vi "Drive Train Motion Track.vi"(6 "Ka":dbl, 7 "PID Settings":T2, 9 "Use Ave":bool, 10 "Array":T1(array[cluster]), 11 "Kv":dbl) -> ()   [LabVIEW 2015]
uses:
  Support/LightningPID Settings.ctl
panel:
  out "Right Velocity Chart":cluster{"left":dbl, "Rate":dbl}(graph)
  out "Right Distance Chart":cluster{"left":dbl, "Rate":dbl}(graph)
  out "Moter Power":cluster{"left":dbl, "Rate":dbl}(graph)
  out "Left Velocity Chart":cluster{"left":dbl, "Rate":dbl}(graph)
  out "Left Distance Chart":cluster{"left":dbl, "Rate":dbl}(graph)
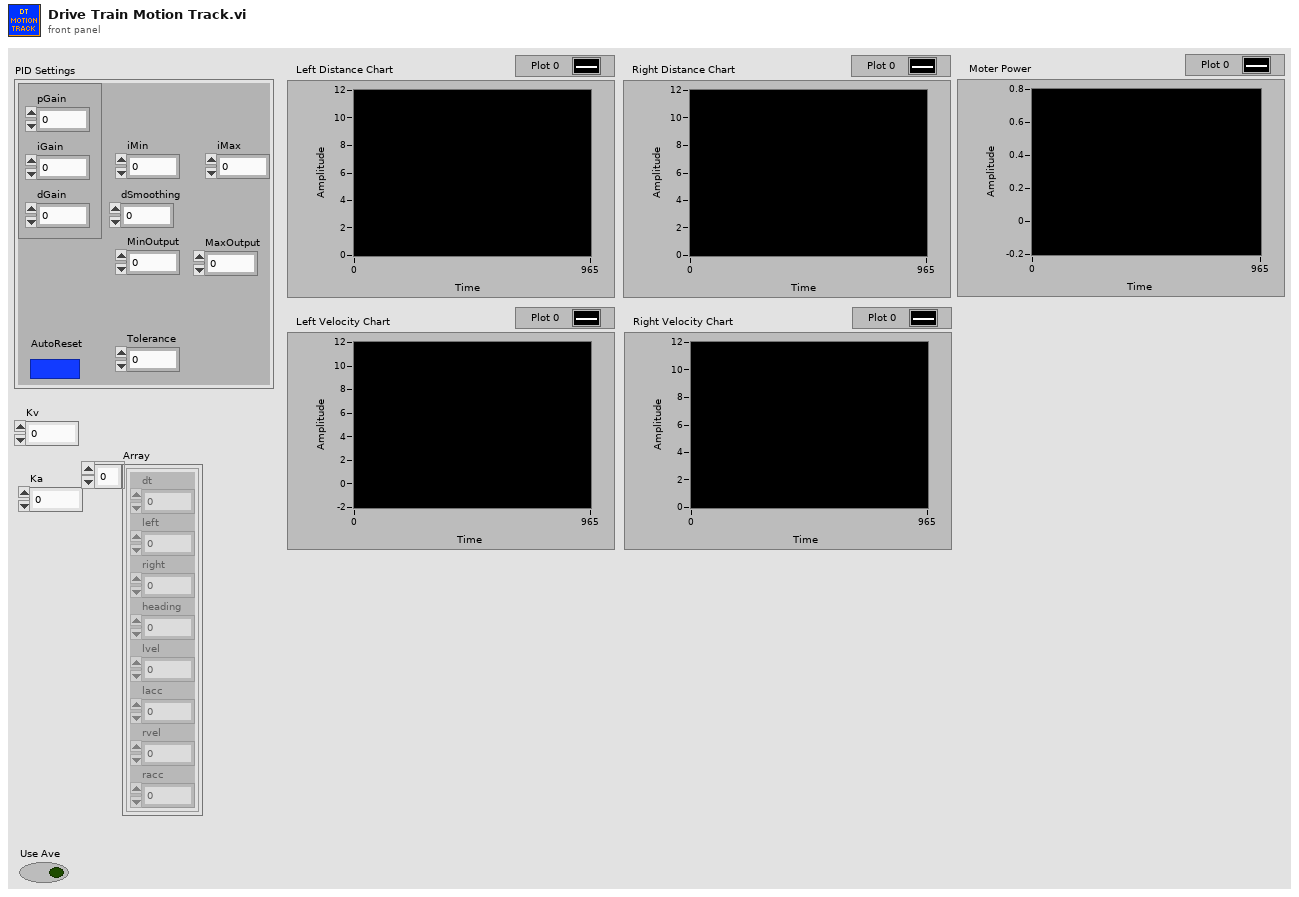
[diagram p1: front panel]
types:
  T1 = cluster{"dt":dbl, "left":dbl, "right":dbl, "heading":dbl, "lvel":dbl, "lacc":dbl, "rvel":dbl, "racc":dbl}[]
  T2 = typedef "LightningPID Settings.ctl" = cluster{"iMax":dbl, "iMin":dbl, "iGain":dbl, "pGain":dbl, "dGain":dbl, "MaxOutput":dbl, "MinOutput":dbl, "AutoReset":bool, "Tolerance":dbl, "dSmoothing":dbl}
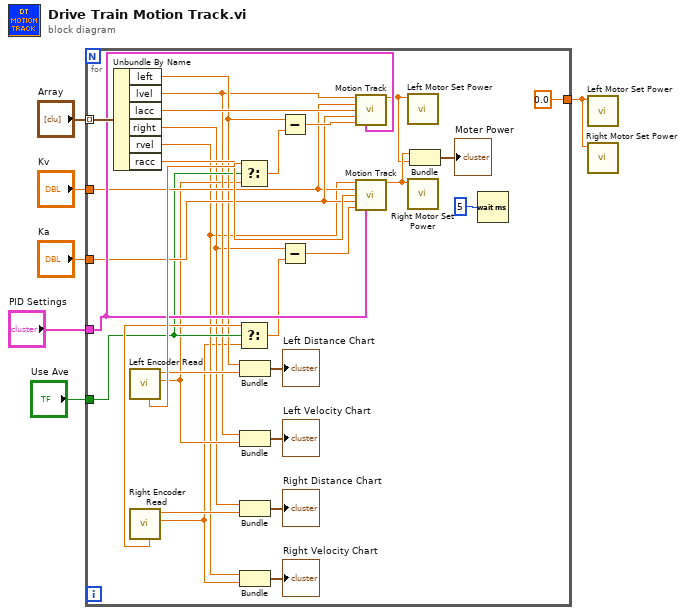
[diagram p0: block diagram]
diagram:
  n1 = for {
    tunnel: "Array" -> [w35] mode=indexing
    tunnel: [0.0] -> w2
    tunnel: "PID Settings" -> [w27]
    tunnel: "Ka" -> [w26]
    tunnel: "Kv" -> [w25]
    tunnel: "Use Ave" -> [w24]
    n2 = Unbundle By Name(w35) -> ("left"=w23:dbl, "lvel"=w20:dbl, "lacc"=w32:dbl, "right"=w12:dbl, "rvel"=w9:dbl, "racc"=w29:dbl)
    n3 = call "Left Encoder Read.vi"() -> ("Rate"=w19:dbl, "Distance"=w21:dbl, "Ave Velocity"=w34:dbl)  [unwired: 7 in, 2 out]
    n4 = call "Right Encoder Read.vi"() -> ("Rate"=w8:dbl, "Distance"=w11:dbl, "Ave Velocity"=w28:dbl)  [unwired: 7 in, 2 out]
    n5 = Select(t=w34, s=w24, f=w19) -> (s? t:f=w31:dbl)
    n6 = Select(t=w28, s=w24, f=w8) -> (s? t:f=w14:dbl)
    n7 = Bundle("left"=w23, "Distance"=w21) -> (→"Left Distance Chart":cluster{"left":dbl, "Distance":dbl})  [unwired: 1 in]
    n8 = Bundle("lvel"=w20, "Rate"=w19) -> (→"Left Velocity Chart":cluster{"lvel":dbl, "Rate":dbl})  [unwired: 1 in]
    n9 = Bundle("right"=w12, "Distance"=w11) -> (→"Right Distance Chart":cluster{"right":dbl, "Distance":dbl})  [unwired: 1 in]
    n10 = Bundle("rvel"=w9, "Rate"=w8) -> (→"Right Velocity Chart":cluster{"rvel":dbl, "Rate":dbl})  [unwired: 1 in]
    n11 = Subtract(x=w23, y=w31) -> (x-y=w30:dbl)
    n12 = Subtract(x=w12, y=w14) -> (x-y=w13:dbl)
    n13 = call "Motion Track.vi"("vel"=w20, "Kv"=w25, "acc"=w32, "Ka"=w26, "error"=w30, "PID Settings"=w27) -> ("Power"=w16:dbl)  [unwired: 9 in]
    n14 = call "Motion Track.vi"("vel"=w9, "Kv"=w25, "acc"=w29, "Ka"=w26, "error"=w13, "PID Settings"=w27) -> ("Power"=w17:dbl)  [unwired: 9 in]
    n15 = call "Left Motor Set Power.vi"("Output"=w16) -> ()  [unwired: 10 in, 1 out]
    n16 = call "Right Motor Set Power.vi"("Output"=w17) -> ()  [unwired: 10 in, 1 out]
    n17 = Bundle("Power"=w17, "Power"=w16) -> (→"Moter Power":cluster{"Power":dbl, "Power":dbl})  [unwired: 1 in]
    n18 = Wait (ms)(milliseconds to wait=u32 5) -> ()  [unwired: 1 out]
  }
  n19 = call "Left Motor Set Power.vi"("Output"=w2) -> ()  [unwired: 10 in, 1 out]
  n20 = call "Right Motor Set Power.vi"("Output"=w2) -> ()  [unwired: 10 in, 1 out]
